vi "Write SelectionMode.vi"(8 "error in (no error)":errorcluster, 10 "Selection Mode":T1, 11 "Msg_Error.lvclass in":refnum<class "ListSelection.lvclass">) -> (0 "error out":errorcluster, 3 "Msg_Error.lvclass out":refnum<class "ListSelection.lvclass">)   [LabVIEW 2012, in "ListSelection.lvlib" / "ListSelection.lvclass"]
uses:
  ListSelection.lvclass
  Selection Mode.ctl
  ListSelection.lvclass/ListSelection.ctl
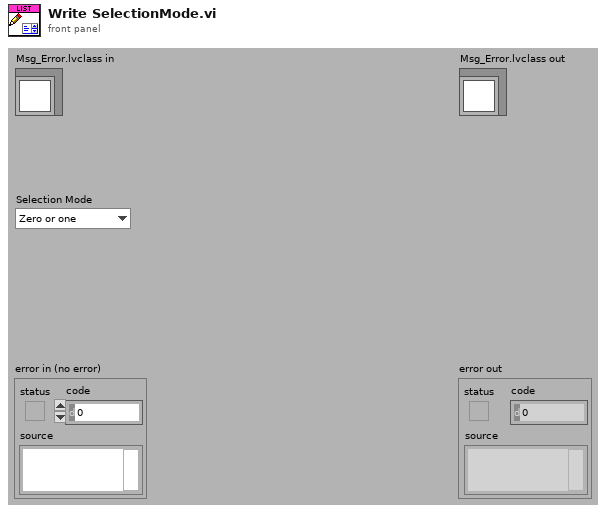
[diagram p1: front panel]
types:
  T1 = typedef "ListSelection.lvlib/ListSelection.lvclass/Selection Mode.ctl" = enum16{"Zero or one", "One", "Zero or more", "One or more"}
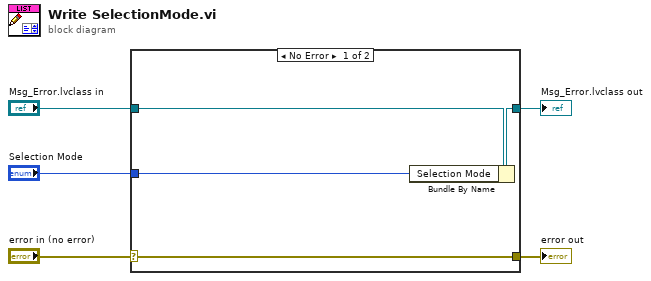
[diagram p0: block diagram]
diagram:
  n1 = case shown="No Error" "error in (no error)" {
    selector: "error in (no error)" -> [w9 w10]
    tunnel: [w9 w10] -> w4
    tunnel: [w7 w11] -> w2
    tunnel: "Msg_Error.lvclass in" -> [w8 w11]
    tunnel: "Selection Mode" -> [w6 _]
    frame No Error {
      n2 = Bundle By Name(cluster=w8, "Selection Mode"=w6) -> (w7:refnum<class "ListSelection.lvclass">)
    }
    frame Error {
    }
  }
  "error out" <- w4
  "Msg_Error.lvclass out" <- w2
